vi "Gaussian Blur.vi"(0 "Image":T1, 5 "Image Dst":T1, 7 "Kernel Size":i32=11, 9 "Standard Deviation":dbl=1.0, 11 "error in":errorcluster) -> (4 "Image Out":T1, 15 "error out":errorcluster)   [LabVIEW 2011]
uses:
  <vilib>/vision/Image Controls.llb/IMAQ Image.ctl
  <vilib>/Analysis/2dsp.llb/2D Convolution (DBL).vi
  <vilib>/Analysis/NI_AALPro.lvlib
  Program Files (x86)/National Instruments/LabVIEW 2011/resource/objmgr/IMAQImage.rc
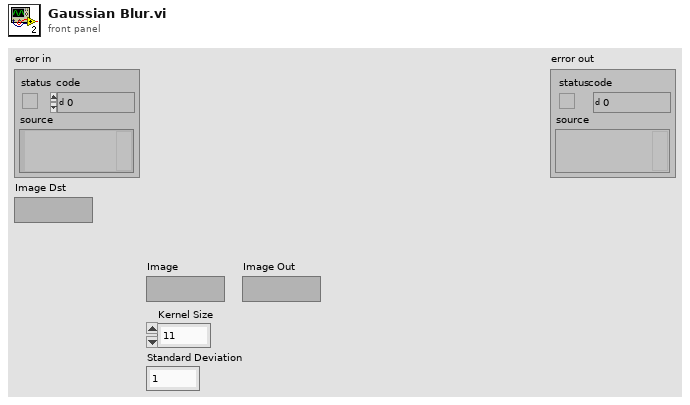
[diagram p1: front panel]
types:
  T1 = typedef "IMAQ Image.ctl" = refnum<image>
  T2 = typedef "Image Type" = u32
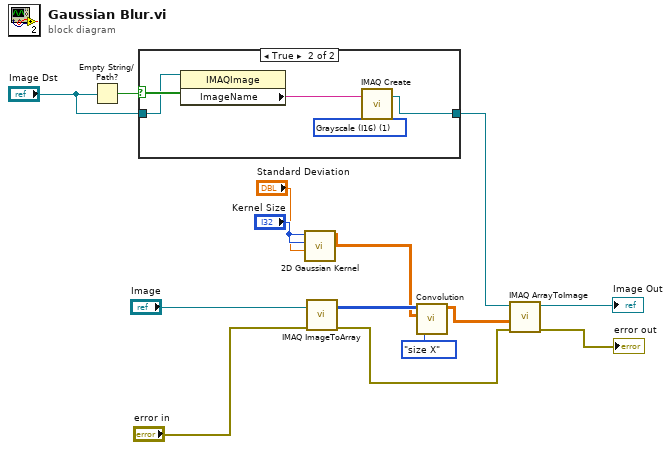
[diagram p0: block diagram]
diagram:
  n1 = Empty String/Path?(string/path="Image Dst") -> (empty?=w4:bool)
  n2 = case shown="True" w4 {
    tunnel: [w15 w18] -> w2
    tunnel: "Image Dst" -> [w15 w16]
    frame False {
    }
    frame True {
      w19 = T2 1 items=["Grayscale (U8)", "Grayscale (I16)", "Grayscale (SGL)", "Complex (CSG)", "RGB (U32)", "HSL (U32)", "RGB (U64)", "Grayscale (U16)"] ("Image Type")
      n3 = property class="IMAQImage"(reference=w16) -> ("ImageName"=w17:string)  [unwired: 1 in, 2 out]
      n4 = call "IMAQ Create"("Image Name"=w17, "Image Type"=w19) -> ("New Image"=w18:T1)  [unwired: 3 in, 1 out]
    }
  }
  n5 = call "2D Gaussian Kernel.vi"("Standard Deviation"="Standard Deviation", "Gaussian Kernel Y Dimension"="Kernel Size", "Gaussian Kernel X Dimension"="Kernel Size") -> ("Kernel"=w11:dbl[][])  [unwired: 8 in]
  n6 = call "IMAQ ImageToArray"("error in (no error)"="error in", "Image"="Image") -> ("error out"=w6:errorcluster, "Image Pixels (I16)"=w12:i16[][])  [unwired: 2 in, 3 out]
  n7 = call-poly <vilib>:"Convolution.vi"("output size"=enum32{"full", "size X", "compact"}."size X", "Y"=w11, "X"=w12) -> ("X * Y"=w9:dbl[][])  [unwired: 7 in, 1 out]
  n8 = call "IMAQ ArrayToImage"("error in (no error)"=w6, "Image Pixels (I16)"=w9, "Image"=w2) -> ("error out"=→"error out":errorcluster, "Image Out"=→"Image Out":T1)  [unwired: 7 in]
